vi "cst--amplitude_units.vi"() -> ()   [LabVIEW 2013]
panel:
  in  "Amplitude Units (ref)":string[](array[string])
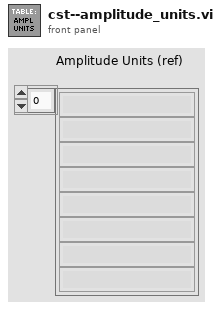
[diagram p1: front panel]
diagram:
